vi "PH_DeformableMirror.GetAllChannels.vi"(0 "VI in":refnum<vi>, 5 "error in (no error)":errorcluster) -> (14 "VI out":refnum<vi>, 19 "error out":errorcluster)   [LabVIEW 2014, in "PH_DeformableMirror.lvlib"]
uses:
  PH_DeformableMirror.lvlib
  instr.lib/dmdriver/DMirrorBase/DMirrorBase.lvclass/DMirrorBase.ctl
  instr.lib/dmdriver/DMirrorBase/DMirrorBase.lvclass
  PH_Common/PH_Common.lvlib
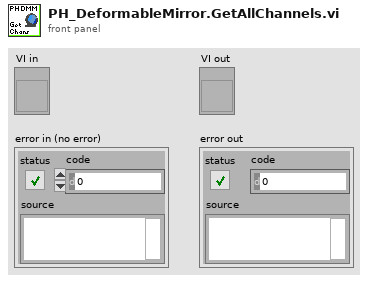
[diagram p1: front panel]
types:
  T1 = typedef "PH_DeformableMirror.lvlib/PH_DeformableMirror.i attribute.ctl" = cluster{"DMirror.lvlib:DMirrorBase.lvclass":refnum<class "DMirrorBase.lvclass">, "Device error":errorcluster, "GUI Refs":cluster{"Delete":refnum<vi>, "Device Error":refnum<vi>, "HV on":refnum<vi>, "Channel":refnum<vi>, "Voltage":refnum<vi>, "Channel Voltages":refnum<vi>}}
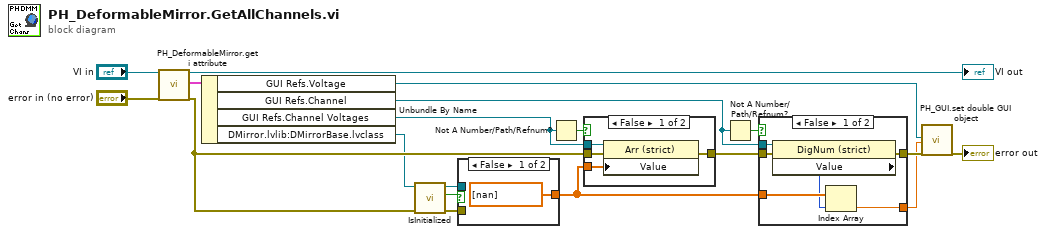
[diagram p0: block diagram]
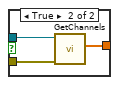
[diagram p2: hidden frame]
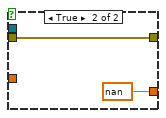
[diagram p3: hidden frame]
diagram:
  n1 = call "PH_DeformableMirror.get i attribute.vi"("i ref in"="VI in", "error in (no error)"="error in (no error)") -> ("i ref out"=→"VI out":refnum<vi>, "i attribute"=w19:T1, "error out"=w5:errorcluster)  [unwired: 15 in]
  n2 = Unbundle By Name(w19) -> ("GUI Refs.Voltage"=w14:refnum<vi>, "GUI Refs.Channel"=w8:refnum<vi>, "GUI Refs.Channel Voltages"=w12:refnum<vi>, "DMirror.lvlib:DMirrorBase.lvclass"=w3:refnum<class "DMirrorBase.lvclass">)
  n3 = call "IsInitialized.vi"("error in (no error)"=w5, "DMirrorBase in"=w3) -> ("error out"=w4:errorcluster, "Initialized?"=w1:bool, "DMirrorBase out"=w2:refnum<class "DMirrorBase.lvclass">)  [unwired: 7 in]
  n4 = case shown="False" w1 {
    tunnel: [dbl[] [nan] ("channel values") w23] -> w7
    tunnel: w4 -> [_ w22]
    tunnel: w2 -> [_ w21]
    frame False {
    }
    frame True {
      n5 = call "GetChannels.vi"("error in (no error)"=w22, "DMirrorBase in"=w21) -> ("channel values"=w23:dbl[])  [unwired: 7 in, 2 out]
    }
  }
  n6 = Not A Number/Path/Refnum?(number/path/refnum=w12) -> (NaN/Path/Refnum?=w13:bool)
  n7 = case shown="False" w13 {
    tunnel: w5 -> [w27 w28]
    tunnel: [w26 w28] -> w10
    tunnel: w12 -> [w25 _]
    tunnel: w7 -> [w24 _]
    frame False {
      n8 = property class="Arr (strict)"(reference=w25, error in=w27, "Value"=w24) -> (error out=w26:errorcluster)  [unwired: 1 out]
    }
    frame True {
    }
  }
  n9 = Not A Number/Path/Refnum?(number/path/refnum=w8) -> (NaN/Path/Refnum?=w11:bool)
  n10 = case shown="False" w11 {
    tunnel: w10 -> [w34 w36]
    tunnel: [w33 w36] -> w9
    tunnel: w8 -> [w32 _]
    tunnel: w7 -> [w31 _]
    tunnel: [w29 nan ("Numeric")] -> w6
    frame False {
      n11 = property class="DigNum (strict)"(reference=w32, error in=w34) -> (error out=w33:errorcluster, "Value"=w30:u32)  [unwired: 1 out]
      n12 = Index Array(array=w31, index=w30) -> (element=w29:dbl)
    }
    frame True {
    }
  }
  n13 = call "PH_GUI.set double GUI object.vi"("GUI object Ref"=w14, "value"=w6, "error in (no error)"=w9) -> ("error out"=→"error out":errorcluster)  [unwired: 16 in]
